vi "square-of-a-number.vi"() -> ()   [LabVIEW 2025]
panel:
  out "x":dbl
  in  "Numeric":dbl
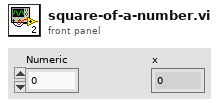
[diagram p1: front panel]
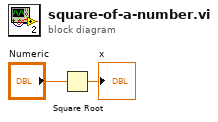
[diagram p0: block diagram]
diagram:
  n1 = Square Root(x="Numeric") -> (sqrt(x)=→"x":dbl)
